vi "Test Filter Test by Name does not Remove Tests on Empty List.vi"(8 "error in (no error)":errorcluster, 11 "Test Case In":refnum<class "Filter Test.lvclass">) -> (0 "error out":errorcluster, 3 "Test Case Out":refnum<class "Filter Test.lvclass">)   [LabVIEW 2020, in "Filter Test.lvclass"]
uses:
  Filter Test.lvclass
  C:/Program Files (x86)/National Instruments/LabVIEW 2020/vi.lib/Astemes/LUnit/Test Case.lvclass
  Test Doubles/Light Test Case Double Copy/Light Test Case Double Copy.lvclass
  <vilib>/Astemes/LUnit/Test Case.lvclass/Test Case.ctl
  c9d5a1b5-bad8-4c9a-9c4d-8f39af3f63be.vi
  <vilib>/Astemes/LUnit/Append Pass Result.vi
  <vilib>/Astemes/LUnit/Append Fail Result.vi
  <vilib>/Astemes/LUnit/Describe Comparison.vi
  <vilib>/Astemes/LUnit/Compare Variants.vi
  <vilib>/Astemes/LUnit/Run In UI.vi
  <vilib>/Utility/error.llb/Clear Errors.vi
  <vilib>/Astemes/LUnit/Describe Variant.vi
  source/User Interface/Support/Filters/Filter/Filter.lvclass
  source/User Interface/Support/Filters/Static Filter/Static Filter.lvclass
  source/API/LUnit Test Suite/LUnit Test Suite.lvclass
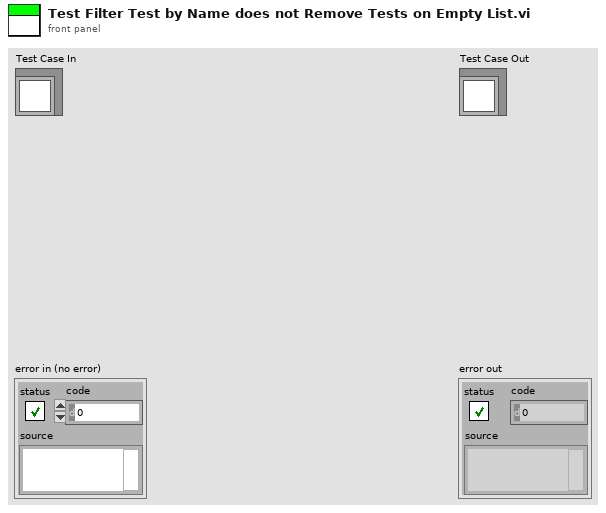
[diagram p1: front panel]
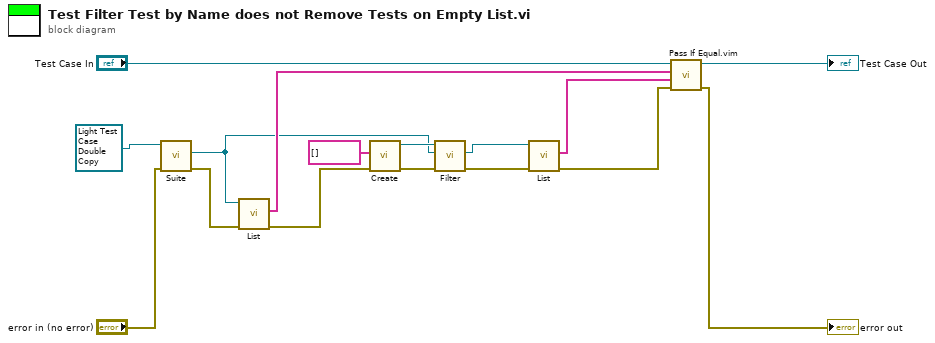
[diagram p0: block diagram]
diagram:
  n1 = call-dynamic "Suite.vi"("error in (no error)"="error in (no error)", "Test Case Class in"=refnum<class "Light Test Case Double Copy.lvclass"> refnum ("Light Test Case Double Copy.lvclass")) -> ("error out"=w12:errorcluster, "LUnit Test Suite Out"=w2:refnum<class "LUnit Test Suite.lvclass">)  [unwired: 7 in, 1 out]
  n2 = call "List.vi"("error in (no error)"=w12, "LUnit Test Suite In"=w2) -> ("error out"=w11:errorcluster, "List of Runnables"=w5:string[])  [unwired: 8 in]
  n3 = call "Create.vi"("error in (no error)"=w11, "Tests"=string[] []) -> ("error out"=w9:errorcluster, "Static Filter"=w10:refnum<class "Filter.lvclass">)  [unwired: 8 in]
  n4 = call-dynamic "Filter.vi"("error in (no error)"=w9, "Test Suite"=w2, "Filter in"=w10) -> ("error out"=w7:errorcluster, "Filtered Test Suite"=w8:refnum<class "LUnit Test Suite.lvclass">)  [unwired: 7 in]
  n5 = call "List.vi"("error in (no error)"=w7, "LUnit Test Suite In"=w8) -> ("error out"=w4:errorcluster, "List of Runnables"=w6:string[])  [unwired: 8 in]
  n6 = call "Pass If Equal.vim"("error in (no error)"=w4, "Actual"=w6, "Expected"=w5, "LUnit Test Case In"="Test Case In") -> ("error out"=→"error out":errorcluster, "LUnit Test Case Out"=→"Test Case Out":refnum<class "Filter Test.lvclass">)  [unwired: 6 in]
